vi "compress_chunk.vi"(7 "connection_reference":T1, 8 "error in (no error)":errorcluster, 10 "if_not_compressed":bool, 11 "chunk_name":string) -> (0 "error out":errorcluster, 3 "compressed_chunk":string)   [LabVIEW 2015, in "lv-timescaledb.lvlib"]
uses:
  lv-timescaledb.lvlib
  <vilib>/addons/database/Connection.llb/Conn ObjectReference.ctl
  <vilib>/addons/database/Command.llb/Cmd Execute.vi
  <vilib>/addons/database/Recordset.llb/Rec Fetch Recordset Data (CR).vi
  <vilib>/addons/database/Recordset.llb/Rec Destroy - Command.vi
  <vilib>/addons/database/Command.llb/Cmd Delete.vi
  <vilib>/addons/database/NI_Database_API.lvlib
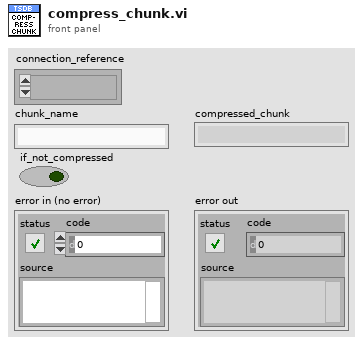
[diagram p1: front panel]
types:
  T1 = typedef "NI_Database_API.lvlib/Conn ObjectReference.ctl" = refnum<k1>
  T2 = cluster{"chunk_name":string, "if_not_compressed":bool}
  T3 = typedef "NI_Database_API.lvlib/DB Tools Parameter Info.ctl" = cluster{"parameter name":string, "type":T4, "direction":T5, "value":variant}
  T4 = typedef "NI_Database_API.lvlib/DB Tools DataTypes.ctl" = enum16{"String", "Long (I32)", "Single (SGL)", "Double (DBL)", "Date/Time", "Binary"}
  T5 = typedef "NI_Database_API.lvlib/DB Tools Parameter Dir.ctl" = enum32{"Input", "Output", "Input/Output", "Return Value"}
  T6 = typedef "NI_Database_API.lvlib/Cmd ObjectReference.ctl" = refnum<k1>
  T7 = typedef "NI_Database_API.lvlib/Cmd-Rec Object Reference.ctl" = refnum<k1>
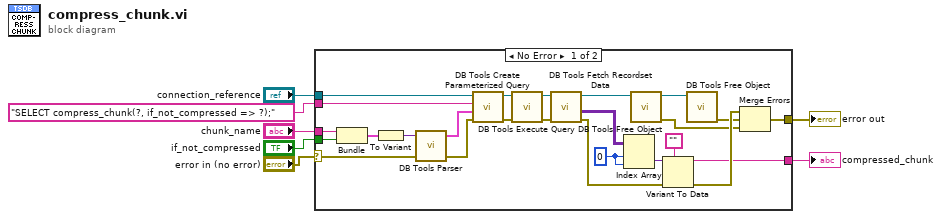
[diagram p0: block diagram]
diagram:
  n1 = case shown="No Error" "error in (no error)" {
    selector: "error in (no error)" -> [w9 w33]
    tunnel: "chunk_name" -> [w19 _]
    tunnel: "connection_reference" -> [w16 _]
    tunnel: [w32 w33] -> w4
    tunnel: [w25 _] -> w1
    tunnel: "SELECT compress_chunk(?, if_not_compressed => ?);" -> [w17 _]
    tunnel: "if_not_compressed" -> [w18 _]
    frame No Error {
      w26 = 0 ("index (row)")
      n2 = Bundle("chunk_name"=w19, "if_not_compressed"=w18) -> (w20:T2)  [unwired: 1 in]
      n3 = To Variant(anything=w20) -> (Variant=w8:variant)
      n4 = call <vilib>:"DB Tools Parser.vi"("error in (no error)"=w9, "variant"=w8) -> ("error out"=w10:errorcluster, "parameters"=w24:T3[])  [unwired: 2 in]
      n5 = call <vilib>:"DB Tools Create Parameterized Query.vi"("error in (no error)"=w10, "parameters"=w24, "SQL query"=w17, "connection reference"=w16) -> ("error out"=w21:errorcluster, "command reference"=w22:T6)  [unwired: 3 in, 1 out]
      n6 = call-poly <vilib>:"DB Tools Execute Query.vi"("error in (no error)"=w21, "command reference"=w22) -> ("error out"=w13:errorcluster, "command-recordset reference"=w15:T7)  [unwired: 6 in]
      n7 = call-poly <vilib>:"DB Tools Fetch Recordset Data.vi"("error in (no error)"=w13, "command-recordset reference"=w15) -> ("error out"=w30:errorcluster, "recordset data"=w28:variant[][], "command-recordset reference out"=w14:T7)  [unwired: 3 in]
      n8 = Index Array(array=w28, index (row)=w26, index (col)=w26) -> (element=w27:variant)
      n9 = call-poly <vilib>:"DB Tools Free Object.vi"("command-recordset reference"=w14) -> ("error out"=w11:errorcluster, "command reference"=w23:T6)  [unwired: 9 in]
      n10 = Variant To Data(error in=w30, type="" ("Array"), Variant=w27) -> (data=w25:string, error out=w29:errorcluster)
      n11 = call-poly <vilib>:"DB Tools Free Object.vi"("command reference"=w23) -> ("error out"=w12:errorcluster)  [unwired: 9 in, 1 out]
      n12 = Merge Errors(w29, w12, w11) -> (w32:errorcluster)
    }
    frame Error {
    }
  }
  "error out" <- w4
  "compressed_chunk" <- w1
